vi "CoMP-S Mechanism - Diffuser Verification.vi"(8 "error in (no error)":errorcluster, 10 "Motors":bool, 11 "Diffuser":T1=enum."In Beam") -> (0 "error out":errorcluster, 3 "Diffuser out":T1=enum."In Beam")   [LabVIEW 2014]
uses:
  Controls/Diffuser.ctl
panel:
  out "String":string
  in  "OK":bool
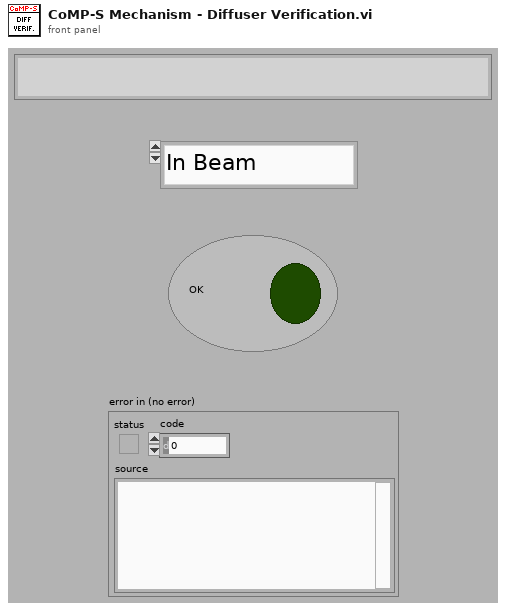
[diagram p1: front panel]
types:
  T1 = typedef "Diffuser.ctl" = enum16{"Out of Beam", "In Beam"}
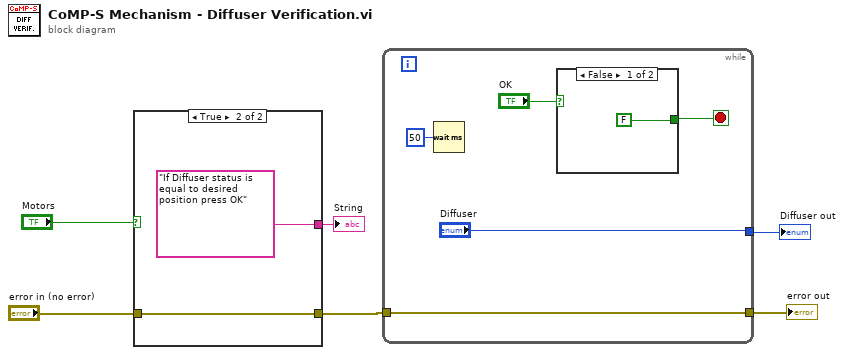
[diagram p0: block diagram]
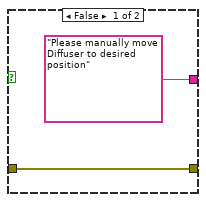
[diagram p2: hidden frame]
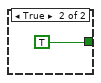
[diagram p3: hidden frame]
diagram:
  n1 = case shown="True" "Motors" {
    tunnel: ["Please manually move Diffuser to desired position" ("String") "If Diffuser status is equal to desired position press OK" ("String")] -> w3
    tunnel: [w8 w9] -> w2
    tunnel: "error in (no error)" -> [w8 w9]
    frame False {
    }
    frame True {
    }
  }
  "String" <- w3
  n2 = while {
    tunnel: w2 -> [w12]
    tunnel: [w12] -> w6
    tunnel: ["Diffuser"] -> w5
    stop <- w13 stop-if-true
    n3 = Wait (ms)(milliseconds to wait=u32 50) -> ()  [unwired: 1 out]
    n4 = case shown="False" "OK" {
      tunnel: [FALSE TRUE] -> w13
      frame False {
      }
      frame True {
      }
    }
  }
  "error out" <- w6
  "Diffuser out" <- w5
